vi "Check 1 module.vi"() -> ()   [LabVIEW 2019]
uses:
  ICPCON ET-7018i/ICPCON ET-7018i.lvclass
  MB_TCP_Timeouts.ctl
  MB_TCP.lvclass/MB_TCP.ctl
  NI_modbus_upd/TCP/TCP.lvclass/TCP.ctl
  ICPCON Status/ICPCON Status.lvlib
  ICPCON Registers/ICPCON Registers.lvlib
  ICPCON Param/ICPCON_Param.lvlib
  MB_TCP.lvclass
panel:
  in  "Start":bool[](array[boolean])
  out "Words out":u16[][](array[numeric])
  out "Connect":bool[](array[boolean])
  in  "stop":bool
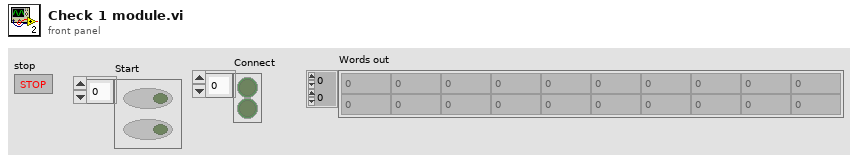
[diagram p1: front panel]
types:
  T1 = typedef "MB_TCP_Timeouts.ctl" = cluster{"reconn_timeout":i32, "N attempt max":i32, "t_reset_TTL":i32, "period":i32}
  T2 = typedef "ICPCON Status.lvlib/ICPCON Status.ctl" = cluster{"Start":refnum<data-value>, "Connect":refnum<data-value>, "WrEn":refnum<data-value>, "IP addr":refnum<data-value>, "Errors":refnum<data-value>, "Stop":refnum<data-value>, "Initialised":bool}
  T3 = cluster{"conn_timeout":i32, "reconn_timeout":i32, "N attempt max":i32, "t_reset_TTL":i32, "write_timeout":i32, "read_timeout":i32, "period":i32}[]
  T4 = cluster{"Remote IP Address":string, "Remote Port":u16}[]
  T5 = typedef "ICPCON Registers.lvlib/ICPCON Data.ctl" = cluster{"UTF":refnum<data-value>, "DI":refnum<data-value>, "DW":refnum<data-value>, "DO":refnum<data-value>, "IR":refnum<data-value>, "WR":refnum<data-value>, "OR":refnum<data-value>, "Initialised":bool}
  T6 = typedef "ICPCON_Param.lvlib/ICPCON Param.ctl" = cluster{"IP addr":refnum<data-value>, "MVIName":refnum<data-value>, "timeouts":refnum<data-value>, "Start":refnum<data-value>, "WR en":refnum<data-value>}
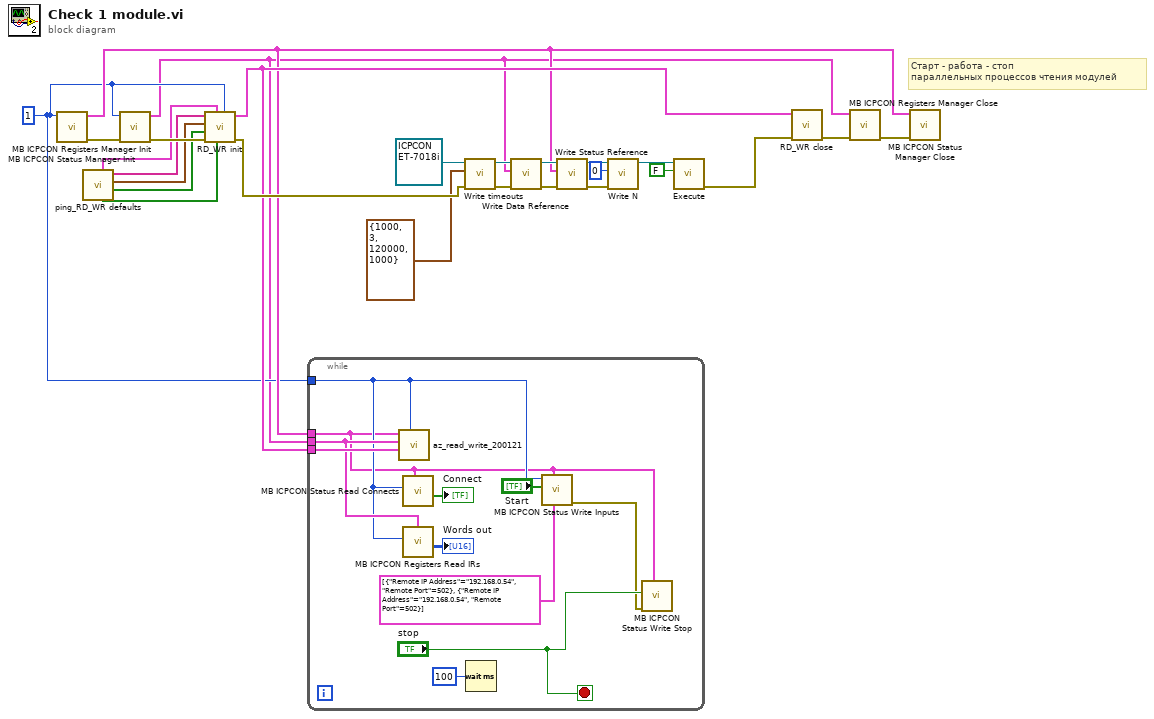
[diagram p0: block diagram]
diagram:
  w4 = 1 ("Data Buffer Length")
  # "Старт - работа - стоп\nпараллельных процессов чтения модулей"
  n1 = call "MB ICPCON Status Manager Init.vi"("Data Buffer Length"=w4) -> ("error out"=w26:errorcluster, "Status Reference"=w5:T2)  [unwired: 9 in]
  n2 = call "ping_RD_WR defaults.vi"() -> ("start def"=w21:bool[], "timeouts def"=w22:T3, "MVIName def"=w23:string[], "WR en def"=w20:bool[], "IP addr def"=w24:T4)  [unwired: 7 in]
  n3 = call "MB ICPCON Registers Manager Init.vi"("error in (no error)"=w26, "Data Buffer Length"=w4) -> ("error out"=w25:errorcluster, "Data Reference"=w3:T5)  [unwired: 8 in]
  n4 = call "RD_WR init.vi"("N_moduls"=w4, "WR en def"=w20, "IP addr def"=w24, "error in"=w25, "start_stop def"=w21, "timeouts def"=w22, "MVIName def"=w23) -> ("error"=w10:errorcluster, "RD_WR param"=w6:T6)  [unwired: 3 in]
  n5 = while {
    tunnel: w6 -> [w37]
    tunnel: w5 -> [w29]
    tunnel: w4 -> [w32]
    tunnel: w3 -> [w35]
    stop <- "stop" stop-if-true
    n6 = call "az_read_write_200121.vi"("N_moduls"=w32, "RD_WR param"=w37, "Data Reference"=w35, "Status Reference"=w29) -> ()  [unwired: 7 in, 1 out]
    n7 = call "MB ICPCON Status Read Connects.vi"("Status Reference"=w29, "Lenght (1)"=w32) -> ("Connect"=→"Connect":bool[])  [unwired: 8 in, 1 out]
    n8 = call "MB ICPCON Registers Read IRs.vi"("Data Reference"=w35, "Length (1)"=w32) -> ("Words out"=→"Words out":u16[][])  [unwired: 8 in, 1 out]
    n9 = Wait (ms)(milliseconds to wait=u32 100) -> ()  [unwired: 1 out]
    n10 = call "MB ICPCON Status Write Inputs.vi"("IP address"=T4 [{"Remote IP Address"="192.168.0.54", "Remote Port"=502}, {"Remote IP Address"="192.168.0.54", "Remote Port"=502}], "Status Reference"=w29, "Start"="Start", "Lenght"=w32) -> ("error out"=w27:errorcluster)  [unwired: 7 in]
    n11 = call "MB ICPCON Status Write Stop.vi"("Status Reference"=w29, "error in (no error)"=w27, "Stop"="stop") -> ()  [unwired: 8 in, 1 out]
  }
  n12 = call "Write timeouts.vi"("error in (no error)"=w10, "timeouts"=T1 {"reconn_timeout"=1000, "N attempt max"=3, "t_reset_TTL"=120000, "period"=1000}, "MB_TCP in"=refnum<class "ICPCON ET-7018i.lvclass"> refnum ("ICPCON ET-7018i.lvclass")) -> ("error out"=w15:errorcluster, "MB_TCP out"=w17:refnum<class "ICPCON ET-7018i.lvclass">)  [unwired: 7 in]
  n13 = call "Write Data Reference.vi"("error in (no error)"=w15, "Data"=w3, "MB_TCP in"=w17) -> ("error out"=w14:errorcluster, "MB_TCP out"=w16:refnum<class "ICPCON ET-7018i.lvclass">)  [unwired: 7 in]
  n14 = call "Write Status Reference.vi"("error in (no error)"=w14, "Status"=w5, "MB_TCP in"=w16) -> ("error out"=w12:errorcluster, "MB_TCP out"=w13:refnum<class "ICPCON ET-7018i.lvclass">)  [unwired: 7 in]
  n15 = call "Write N.vi"("error in (no error)"=w12, "N"=0, "MB_TCP in"=w13) -> ("MB_TCP out"=w8:refnum<class "ICPCON ET-7018i.lvclass">)  [unwired: 7 in, 1 out]
  n16 = call "Execute.vi"("stop"=FALSE, "MB_TCP in"=w8) -> ("error out"=w7:errorcluster)  [unwired: 7 in, 2 out]
  n17 = call "RD_WR close.vi"("error in"=w7, "RD_WR param"=w6) -> ("error out"=w19:errorcluster)  [unwired: 9 in]
  n18 = call "MB ICPCON Registers Manager Close.vi"("error in"=w19, "Data Reference"=w3) -> ("error out"=w18:errorcluster)  [unwired: 9 in]
  n19 = call "MB ICPCON Status Manager Close.vi"("error in"=w18, "Status Reference"=w5) -> ()  [unwired: 9 in, 1 out]
